vi "Shooter Elevation Positons.vi"() -> ()   [LabVIEW 2012]
panel:
  in  "Competiton Climber Home":dbl=0.48
  in  "Climber Home":dbl=0.2
  in  "Bar Home":dbl=2.5
  in  "Competition Extender":dbl
  in  "Competition Winch up":dbl=4.9
  in  "Competition Counterbalance up":dbl=2.1
  in  "Competition Start Elevator":dbl=0.3
  in  "Counterbalance up":dbl=4.95
  in  "Counterbalance down":dbl=3.92
  in  "Climb Elevator":dbl=4.0
  in  "Start  Elevator":dbl=1.73
  in  "Feeder Station Elevation":dbl=3.4
  in  "Elevation Low":dbl=3.3
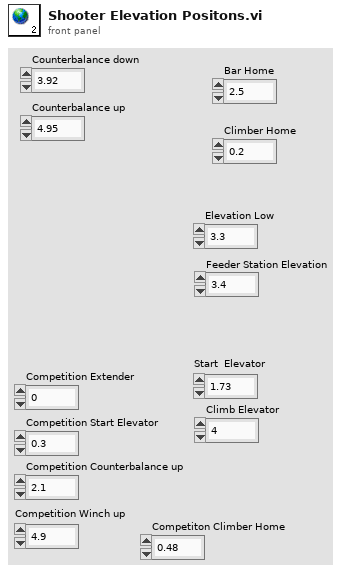
[diagram p1: front panel]
diagram:
